vi "struct_ads_sur_dp_dw_wT.vi"(8 "Error (Input)":errorcluster, 9 "Temperature in K (input)":dbl, 10 "Loading in kg/kg (Input)":dbl, 11 "Reference working pair (Input)":i64) -> (0 "Error (Output)":errorcluster caption="Error(Output)", 3 "Der. pressure wrt. loading in Pakg/kg (Output)":dbl)   [LabVIEW 2017]
doc: "ads_sur_dp_dw_wT:\n * -----------------\n *\n * Calculates derivative of equilibrium pressure p with respect to loading\n * w in kgPa/kg depending on equilibrium loading w in kg/kg and equilibrium\n * temperature T in K.\n *\n * Parameters:\n * -----------\n * double w_kgkg:\n * Equilibrium loading in kg/kg.\n * double T_K:\n * Equilibrium temperature in K.\n * struct *WorkingPair:\n * Pointer of WorkingPair-struct.\n *\n * Returns:\n * --------\n * double:\n * Derivative of equilibrium pressure wrt. loading in Pakg/kg.\n *\n * Remarks:\n * --------\n * This function is only valid for isotherm models based on the surface\n * approach.\n *\n * History:\n * --------\n * 07/13/2021, by Jannik Driesel (supervised by Mirko Engelpracht):\n * First implementation."
uses:
  data/win32bit/libsorpPropLib.dll
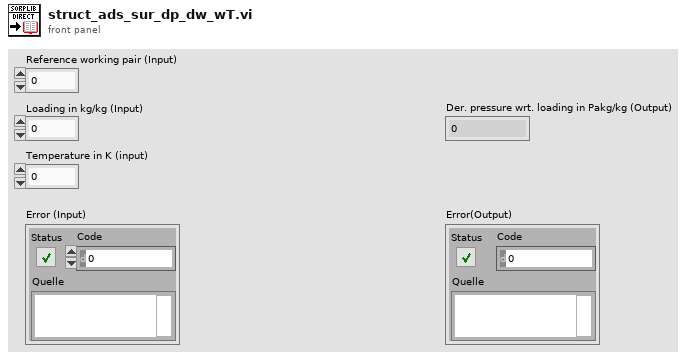
[diagram p1: front panel]
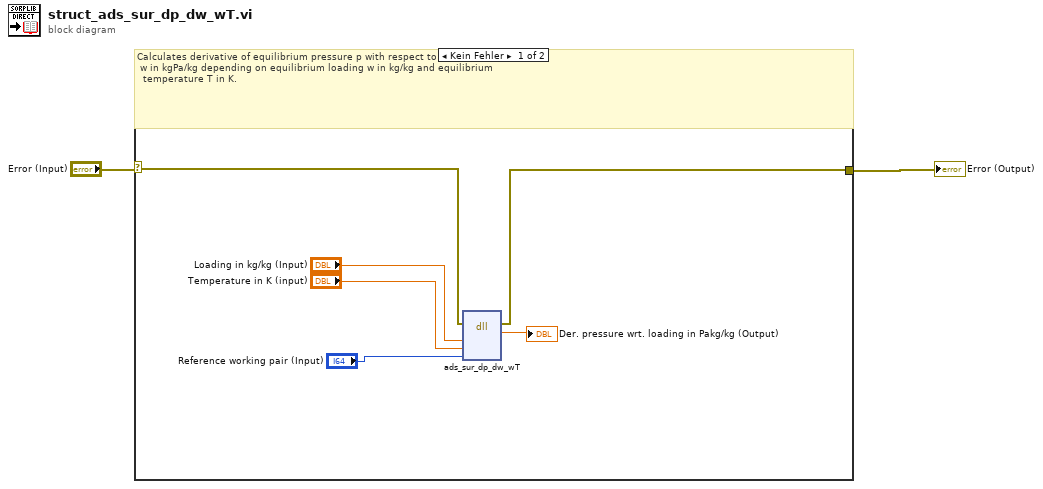
[diagram p0: block diagram]
diagram:
  n1 = case shown="Kein Fehler" "Error (Input)" {
    selector: "Error (Input)" -> [w7 w9]
    tunnel: [w6 w9] -> w1
    frame No Error {
      # "Calculates derivative of equilibrium pressure p with respect to loading\n w in kgPa/kg depending on equilibrium loading w in kg/kg and equilibrium\n  temperature T in K."
      n2 = dll-call lib="D:/Driesel/SorpLibLocal/LabVIEW_wrapper/data/win32bit/libsorpPropLib.dll" fn="ads_sur_dp_dw_wT"(error in=w7, "w_kgkg"="Loading in kg/kg (Input)", "T_K"="Temperature in K (input)", "workingPair"="Reference working pair (Input)") -> (error out=w6:errorcluster, "dp_dw_Pakgkg"=→"Der. pressure wrt. loading in Pakg/kg (Output)":dbl)  [unwired: 5 in, 1 out]
    }
    frame Error {
      # "Error - No calculations"
    }
  }
  "Error (Output)" <- w1
